vi "Sending_TestMode_Recipe_With_TestMode_Cmd_SUB_VI.vi"(0 "Socket IP Address":string="192.168.1.100", 1 "Socket Port Number":u16=1600, 2 "Receipe Msg ID":i32=65, 3 "Receipe Message length":i32=36, 4 "Response ID":u8=66, 5 "error in (no error)":errorcluster, 6 "TestAmplitudeLoopC1":i32=500, 7 "TestFrequencyHigh":i32=500, 8 "TestAmplitudeLoopC2":i32=100, 9 "TestFrequencyLow":i32=450, 10 "TestPhaseLoopI":i32=300, 11 "TestAmplitude":i32=450, 12 "TestPhaseLoopCF":i32=500) -> (16 "Test Mode Signature":string, 19 "error out":errorcluster)   [LabVIEW 2017]
panel:
  out "connection ID out":refnum<k5>
  # "INPUT :"
  # "INFO :"
  # "Parameter Name                                        20KHz                                                                                                          \t40KHz\t\t\n\t                                        Default Value\t    Min Value\t       Max Value\t                                     Default Value         \tMin Value\t            Max Value\nTestAmplitudeLoopC1   100                         1                        20000                                               205                            1                             20000\nTestAmplitudeLoopC2   300                         1                        20000                                               370                            1                             20000\nTestPhaseLoopI               450                         50                      500                                                   60                             50                               500\nTestPhaseLoopCF           450                         50                       500                                                  200                           50                               500\nTestFrequencyHigh        20450                   Note                    Note                                                40900                      Note                           Note\nTestFrequencyLow          19450                   Note                   Note                                                38900                       Note                           Note\nTestAmplitude                 50                           10                       100                                                  50                             10                                100\n\nNote:  FreqLow and FreqHigh cannot cross and must remain within the band"
  # "OUTPUT :"
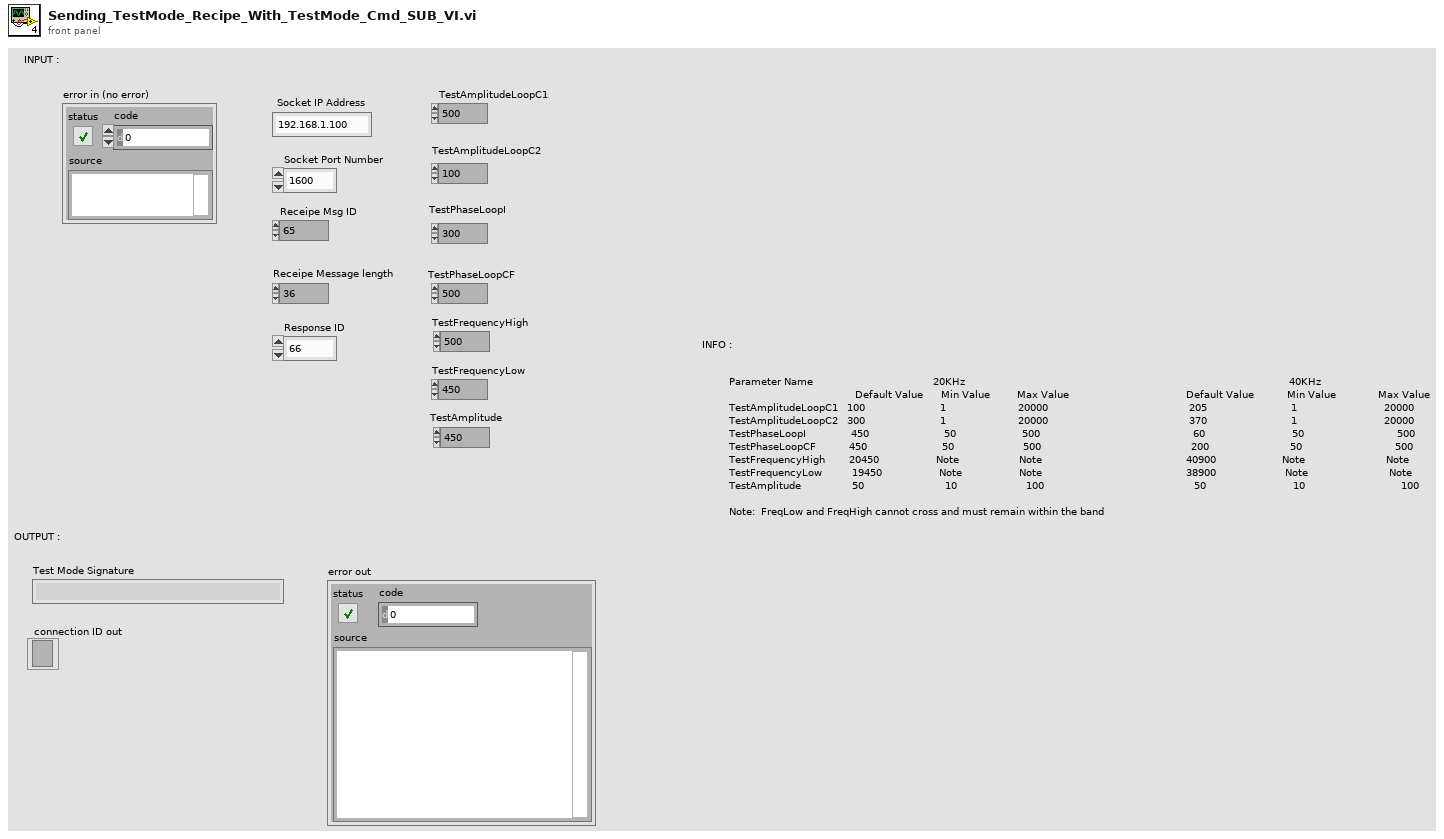
[diagram p1: front panel]
types:
  T1 = enum16{"Standard", "Buffered", "CRLF", "Immediate"}
  T2 = cluster{"Test mode Request Message Length to DB ":i32, "Test mode Request Message ID to DB":i32}
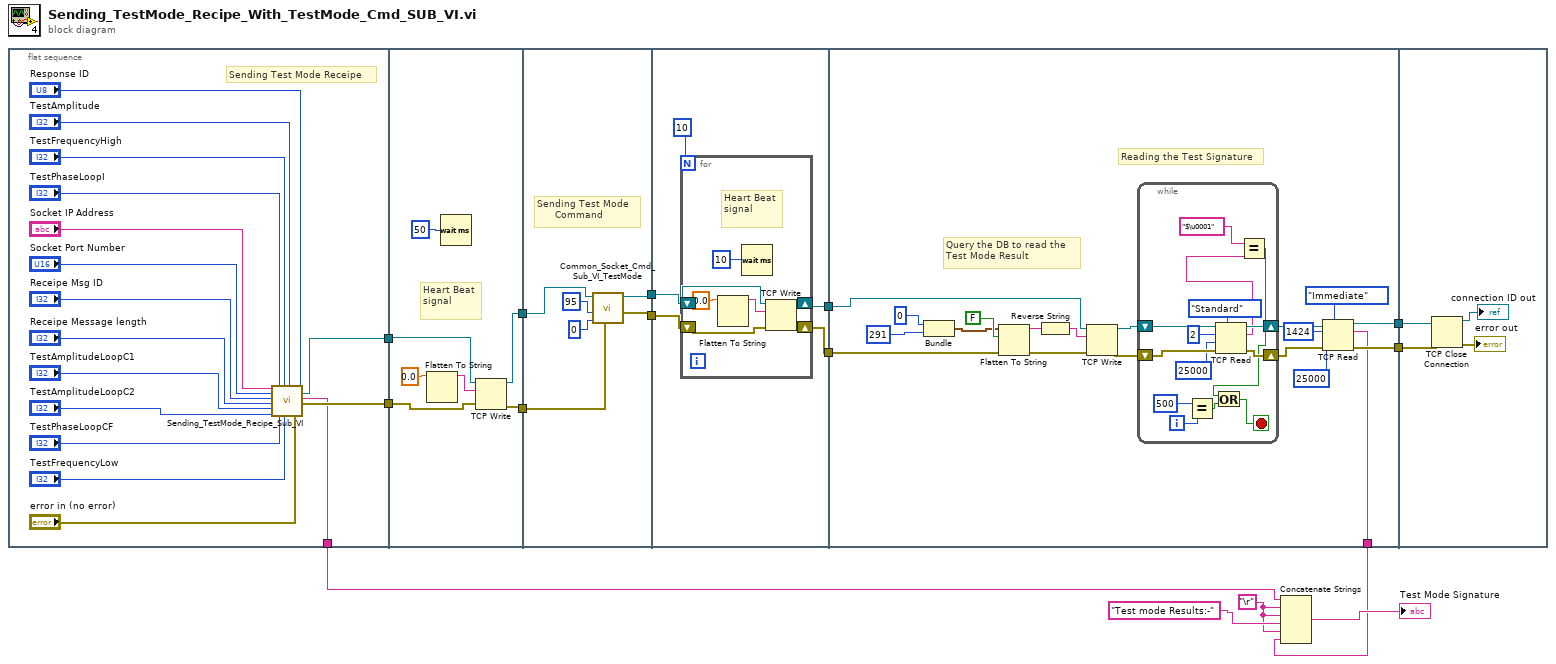
[diagram p0: block diagram]
diagram:
  w2 = "\r"
  n1 = flat-sequence {
    tunnel: [w31] -> w15
    tunnel: [w30] -> w14
    tunnel: [w16] -> w6
    tunnel: w15 -> [w37]
    tunnel: w14 -> [w36]
    tunnel: [w34] -> w13
    tunnel: [w35] -> w12
    tunnel: w13 -> [w44]
    tunnel: w12 -> [w43]
    tunnel: [w42] -> w11
    tunnel: [w41] -> w10
    tunnel: w11 -> [w48]
    tunnel: w10 -> [w49]
    tunnel: [w47] -> w9
    tunnel: [w46] -> w8
    tunnel: w9 -> [w68]
    tunnel: w8 -> [w67]
    tunnel: [w63] -> w5
    tunnel: [w61] -> w4
    tunnel: [w57] -> w1
    tunnel: w5 -> [w91]
    tunnel: w4 -> [w90]
    frame #0 {
      # "Sending Test Mode Receipe"
      n2 = call "Sending_TestMode_Recipe_Sub_VI.vi"("Socket IP Address"="Socket IP Address", "Socket Port Numeber"="Socket Port Number", "Receipe Msg ID"="Receipe Msg ID", "Receipe Message length"="Receipe Message length", "TestAmplitudeLoopC1"="TestAmplitudeLoopC1", "TestAmplitudeLoopC2"="TestAmplitudeLoopC2", "TestPhaseLoopI"="TestPhaseLoopI", "TestPhaseLoopCF"="TestPhaseLoopCF", "TestFrequencyHigh"="TestFrequencyHigh", "TestFrequencyLow"="TestFrequencyLow", "TestAmplitude"="TestAmplitude", "error in (no error)"="error in (no error)", "Response ID"="Response ID") -> ("connection ID"=w31:refnum<k5>, "Test Mode recipe parameters \nRange validation"=w16:string, "error output"=w30:errorcluster)  [unwired: 4 in]
    }
    frame #1 {
      # "Heart Beat \nsignal"
      n3 = Flatten To String(anything=0.0) -> (data string=w32:string)  [unwired: 3 in, 2 out]
      n4 = Wait (ms)(milliseconds to wait=u32 50) -> ()  [unwired: 1 out]
      n5 = TCP Write(connection ID=w37, data in=w32, error in (no error)=w36) -> (connection ID out=w34:refnum<k5>, error out=w35:errorcluster)  [unwired: 1 in, 1 out]
    }
    frame #2 {
      # "Sending Test Mode\n      Command"
      n6 = call "Common_Socket_Cmd_Sub_VI_TestMode.vi"("Common Socket Error in"=w43, "Operation Message Length"=0 ("Operation Message Length 1"), "Operation Message ID"=95 ("Operation Message ID 1"), "connection ID"=w44) -> ("error output"=w42:errorcluster, "connection ID"=w41:refnum<k5>)  [unwired: 6 in]
    }
    frame #3 {
      n7 = for {
        N: 10 -> [_]
        shift-right: [w51] -> w47
        shift-left: w49 -> [w54]
        shift-right: [w50] -> w46
        shift-left: w48 -> [w53]
        # "Heart Beat \nsignal"
        n8 = Flatten To String(anything=0.0) -> (data string=w55:string)  [unwired: 3 in, 2 out]
        n9 = Wait (ms)(milliseconds to wait=u32 10) -> ()  [unwired: 1 out]
        n10 = TCP Write(connection ID=w54, data in=w55, error in (no error)=w53) -> (connection ID out=w51:refnum<k5>, error out=w50:errorcluster)  [unwired: 1 in, 1 out]
      }
    }
    frame #4 {
      # "Query the DB to read the \nTest Mode Result"
      # "Reading the Test Signature"
      n11 = Bundle("Test mode Request Message Length to DB"=0, "Test mode Request Message ID to DB"=291) -> (w69:T2)  [unwired: 1 in]
      n12 = Flatten To String(anything=w69, prepend array or string size? (T)=FALSE, error in (no error)=w67) -> (data string=w75:string, error out=w73:errorcluster)  [unwired: 1 in, 1 out]
      n13 = Reverse String(1:w75) -> (0:w74:string)
      n14 = TCP Write(connection ID=w68, data in=w74, error in (no error)=w73) -> (connection ID out=w66:refnum<k5>, error out=w65:errorcluster)  [unwired: 1 in, 1 out]
      n15 = while {
        shift-right: [w87] -> w64
        shift-left: w66 -> [w89]
        shift-right: [w86] -> w62
        shift-left: w65 -> [w88]
        i -> [w82]
        stop <- w79 stop-if-true
        n16 = Equal?(x=500, y=w82) -> (x = y?=w80:bool)
        n17 = TCP Read(connection ID=w89, bytes to read=2, error in (no error)=w88, 7:T1."Standard" ("mode (standard)"), 9:25000 ("timeout ms (25000)")) -> (connection ID out=w87:refnum<k5>, data out=w77:string, error out=w86:errorcluster)
        n18 = Equal?(x="$\u0001", y=w77) -> (x = y?=w78:bool)
        n19 = Or(x=w78, y=w80) -> (x .or. y?=w79:bool)
      }
      n20 = TCP Read(connection ID=w64, bytes to read=1424, error in (no error)=w62, 7:T1."Immediate" ("mode (standard)"), 9:25000 ("timeout ms (25000)")) -> (connection ID out=w63:refnum<k5>, data out=w57:string, error out=w61:errorcluster)
    }
    frame #5 {
      n21 = TCP Close Connection(connection ID=w91, error in (no error)=w90) -> (connection ID out=→"connection ID out":refnum<k5>, error out=→"error out":errorcluster)  [unwired: 1 in]
    }
  }
  n22 = Concatenate Strings(w6, w2, w2, "Test mode Results:-", w2, w1) -> (→"Test Mode Signature":string)
